vi "Plot_FFID_Calibs.vi"() -> ()   [LabVIEW 2022 SP3]
panel:
  out "Plot 6":string
  out "Plot 5":string
  out "Plot 4":string
  out "Plot 3":string
  out "Plot 2":string
  out "Plot 1":string
  out "Calib 4":cluster{dbl[], dbl[]}[](graph)
  out "Calib 5":cluster{dbl[], dbl[]}[](graph)
  out "Calib 2":cluster{dbl[], dbl[]}[](graph)
  out "Zero":cluster{dbl[], dbl[]}[](graph)
  out "Calib 1":cluster{dbl[], dbl[]}[](graph)
  in  "History (days)":i32=5 min=0
  out "Calib 3":cluster{dbl[], dbl[]}[](graph)
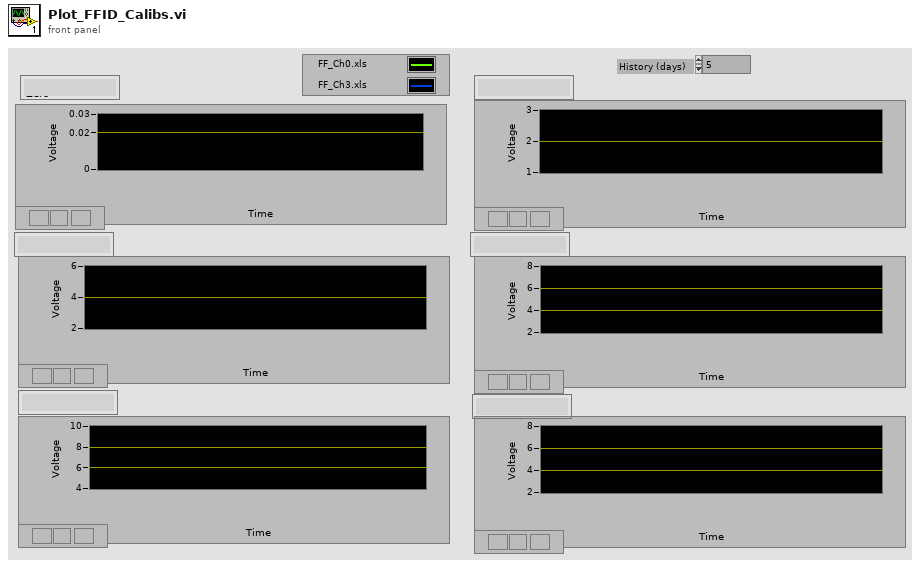
[diagram p1: front panel]
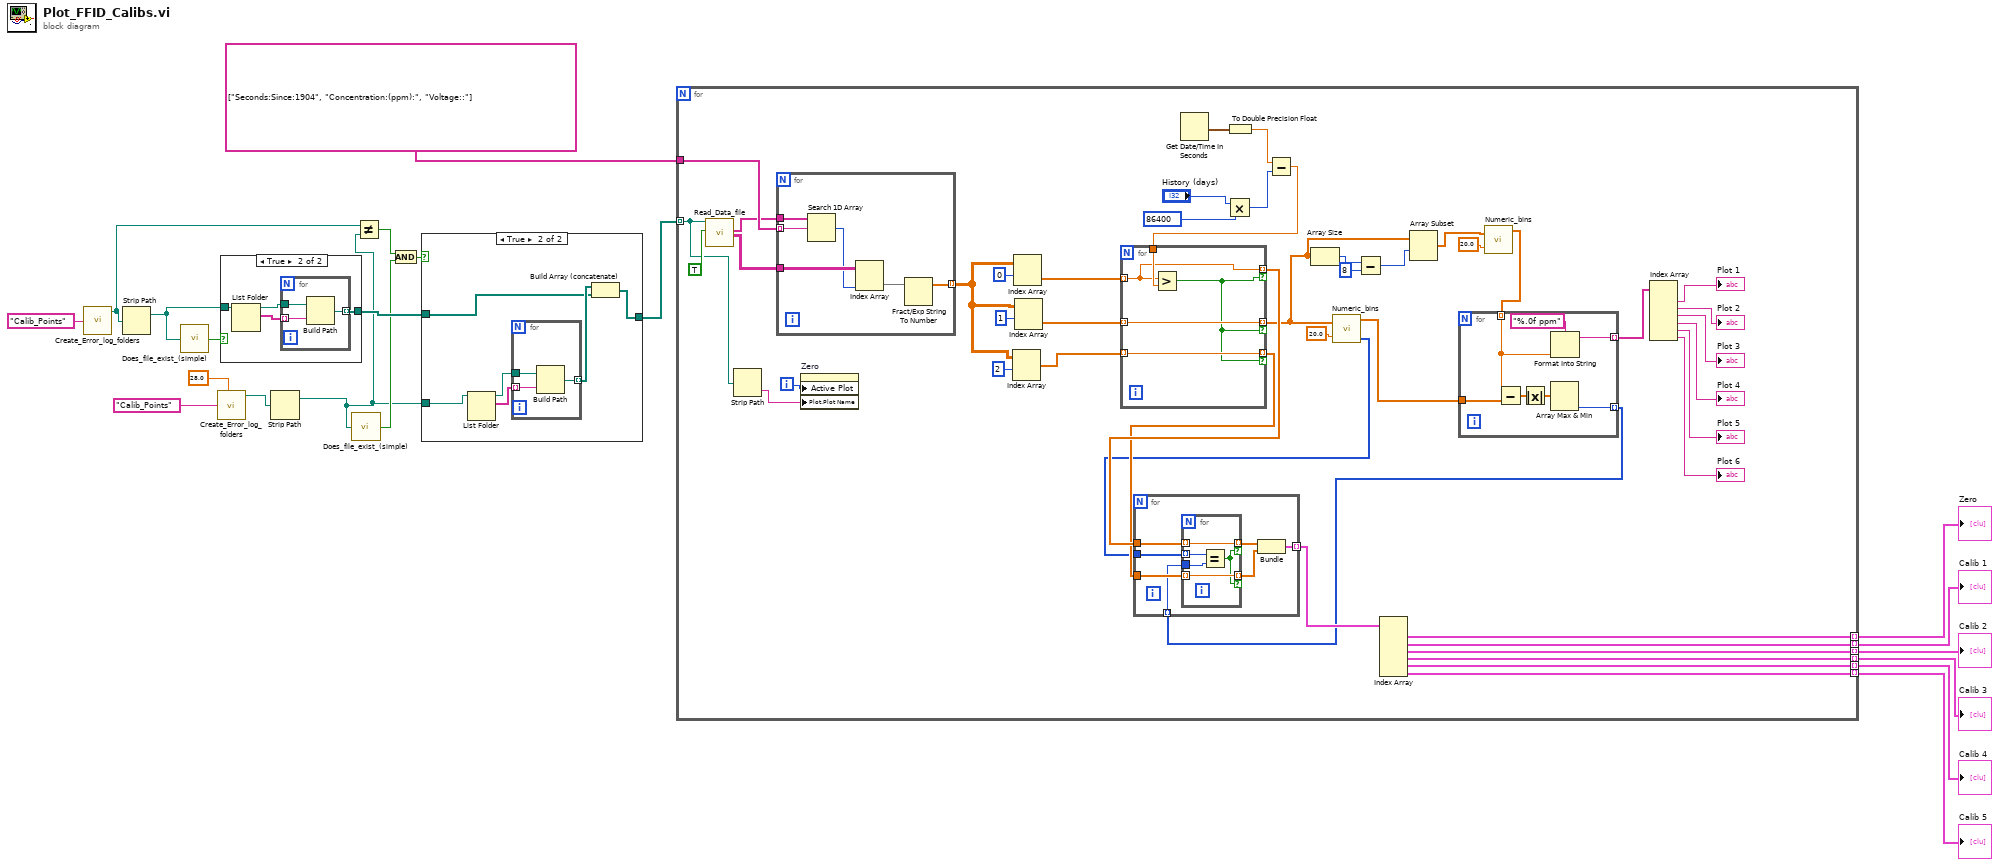
[diagram p0: block diagram]
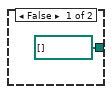
[diagram p2: hidden frame]
diagram:
  n1 = call "Create_Error_log_folders.vi"("Log Folder"="Calib_Points") -> ("Local Log File"=w2:path)  [unwired: 5 in, 1 out]
  n2 = Strip Path(path=w2) -> (stripped path=w16:path)  [unwired: 1 out]
  n3 = call "Does_file_exist_(simple).vi"("Pathname"=w16) -> ("exists?"=w15:bool)
  n4 = call "Create_Error_log_folders.vi"("Days ago"=28.0, "Log Folder"="Calib_Points") -> ("Local Log File"=w1:path)  [unwired: 4 in, 1 out]
  n5 = case shown="True" w15 {
    tunnel: [path[] [] w23] -> w17
    tunnel: w16 -> [_ w22]
    frame False {
    }
    frame True {
      n6 = List Folder(path=w22) -> (path out=w25:path, filenames=w24:string[])  [unwired: 3 in, 2 out]
      n7 = for {
        tunnel: w25 -> [w28]
        tunnel: w24 -> [w27] mode=indexing
        tunnel: [w26] -> w23 mode=indexing
        n8 = Build Path(base path=w28, name or relative path=w27) -> (appended path=w26:path)
      }
    }
  }
  n9 = Strip Path(path=w1) -> (stripped path=w11:path)  [unwired: 1 out]
  n10 = call "Does_file_exist_(simple).vi"("Pathname"=w11) -> ("exists?"=w12:bool)
  n11 = Not Equal?(x=w2, y=w11) -> (x != y?=w14:bool)
  n12 = And(x=w14, y=w12) -> (x .and. y?=w13:bool)
  n13 = case shown="True" w13 {
    tunnel: w11 -> [_ w32]
    tunnel: w17 -> [w29 w30]
    tunnel: [w29 w33] -> w5
    frame False {
    }
    frame True {
      n14 = List Folder(path=w32) -> (path out=w35:path, filenames=w34:string[])  [unwired: 3 in, 2 out]
      n15 = for {
        tunnel: w35 -> [w38]
        tunnel: w34 -> [w37] mode=indexing
        tunnel: [w36] -> w31 mode=indexing
        n16 = Build Path(base path=w38, name or relative path=w37) -> (appended path=w36:path)
      }
      n17 = Build Array (concatenate)(w31, w30) -> (w33:path[])
    }
  }
  n18 = for {
    tunnel: string[] ["Seconds:Since:1904", "Concentration:(ppm):", "Voltage::"] ("Ch names Out") -> [w84]
    tunnel: [w70] -> w9 mode=indexing
    tunnel: [w69] -> w8 mode=indexing
    tunnel: [w68] -> w7 mode=indexing
    tunnel: [w67] -> w6 mode=indexing
    tunnel: w5 -> [w41] mode=indexing
    tunnel: [w57] -> w4 mode=indexing
    tunnel: [w56] -> w3 mode=indexing
    i -> [w39]
    n19 = call "Read_Data_file.vi"("Results file"=w41, "Delete First Rows?"=TRUE) -> ("Ch names Out"=w44:string[], "Channel Values Out"=w43:string[][])  [unwired: 8 in, 8 out]
    n20 = Strip Path(path=w41) -> (name=w40:string)  [unwired: 1 out]
    n21 = for {
      tunnel: w44 -> [w91]
      tunnel: w84 -> [w90] mode=indexing
      tunnel: w43 -> [w89]
      tunnel: [w86] -> w45 mode=indexing
      n22 = Search 1D Array(1D array=w91, element=w90) -> (index of element=w87:i32)  [unwired: 1 in]
      n23 = Index Array(array=w89, index (col)=w87) -> (element=w88:string[])  [unwired: 1 in]
      n24 = Fract/Exp String To Number(string=w88) -> (number=w86:dbl[])  [unwired: 3 in, 1 out]
    }
    n25 = property on="Zero" class="XYGraph (strict)"("Active Plot"=w39, "Plot.Plot Name"=w40) -> ()  [unwired: 2 in, 2 out]
    n26 = Index Array(array=w45, index (row)=2) -> (element=w73:dbl[])  [unwired: 1 in]
    n27 = Index Array(array=w45, index (row)=0) -> (element=w76:dbl[])  [unwired: 1 in]
    n28 = Index Array(array=w45, index (row)=1) -> (element=w74:dbl[])  [unwired: 1 in]
    n29 = Get Date/Time In Seconds() -> (seconds since 1Jan1904=w82:timestamp)
    n30 = Multiply(x="History (days)", y=86400) -> (x*y=w78:i32)
    n31 = To Double Precision Float(number=w82) -> (double precision float=w79:dbl)
    n32 = Subtract(x=w79, y=w78) -> (x-y=w77:dbl)
    n33 = for {
      tunnel: w76 -> [w102] mode=indexing
      tunnel: w77 -> [w103]
      tunnel: [w102] -> w75 mode=indexing if=w99
      tunnel: [w101] -> w65 mode=indexing if=w99
      tunnel: w74 -> [w101] mode=indexing
      tunnel: [w100] -> w72 mode=indexing if=w99
      tunnel: w73 -> [w100] mode=indexing
      n34 = Greater?(x=w102, y=w103) -> (0:w99:bool)
    }
    n35 = Array Size(array=w65) -> (size(s)=w64:i32)
    n36 = call "Numeric_bins.vi"("Values"=w65, "Tolerance"=20.0) -> ("Bin Centres"=w60:dbl[], "Bin Index"=w71:i32[])  [unwired: 1 out]
    n37 = Subtract(x=w64, y=8) -> (x-y=w62:i32)
    n38 = Array Subset(array=w65, index=w62) -> (w61:dbl[])  [unwired: 1 in]
    n39 = call "Numeric_bins.vi"("Values"=w61, "Tolerance"=20.0) -> ("Bin Centres"=w58:dbl[])  [unwired: 2 out]
    n40 = for {
      tunnel: w58 -> [w94] mode=indexing
      tunnel: w60 -> [w98]
      tunnel: [w97] -> w59 mode=indexing
      tunnel: [w92] -> w55 mode=indexing
      n41 = Subtract(x=w94, y=w98) -> (x-y=w96:dbl[])
      n42 = Absolute Value(x=w96) -> (abs(x)=w95:dbl[])
      n43 = Array Max & Min(array=w95) -> (min index (indices)=w97:i32)  [unwired: 3 out]
      n44 = Format Into String(format string="%.0f ppm", w94) -> (resulting string=w92:string)  [unwired: 2 in, 1 out]
    }
    n45 = for {
      tunnel: w71 -> [w110]
      tunnel: w75 -> [w107]
      tunnel: w72 -> [w106]
      tunnel: [w105] -> w85 mode=indexing
      tunnel: w59 -> [w104] mode=indexing
      n46 = for {
        tunnel: w104 -> [w115]
        tunnel: w110 -> [w114] mode=indexing
        tunnel: [w113] -> w109 mode=indexing if=w111
        tunnel: w106 -> [w113] mode=indexing
        tunnel: [w112] -> w108 mode=indexing if=w111
        tunnel: w107 -> [w112] mode=indexing
        n47 = Equal?(x=w114, y=w115) -> (x = y?=w111:bool)
      }
      n48 = Bundle(w108, w109) -> (w105:cluster{dbl[], dbl[]})  [unwired: 1 in]
    }
    n49 = Index Array(array=w85) -> (element #1=w70:cluster{dbl[], dbl[]}, element #2=w69:cluster{dbl[], dbl[]}, element #3=w68:cluster{dbl[], dbl[]}, element #4=w67:cluster{dbl[], dbl[]}, element #5=w57:cluster{dbl[], dbl[]}, element #6=w56:cluster{dbl[], dbl[]})  [unwired: 6 in]
    n50 = Index Array(array=w55) -> (element #1=→"Plot 1":string, element #2=→"Plot 2":string, element #3=→"Plot 3":string, element #4=→"Plot 4":string, element #5=→"Plot 5":string, element #6=→"Plot 6":string)  [unwired: 6 in]
  }
  "Calib 3" <- w6
  "Calib 1" <- w8
  "Zero" <- w9
  "Calib 2" <- w7
  "Calib 5" <- w3
  "Calib 4" <- w4
